vi "LoadState.vi"(3 "tabs":refnum<vi>, 4 "camera":string, 5 "file":path) -> ()   [LabVIEW 2010]
uses:
  <vilib>/addons/h5labview/H5F_mode.ctl
  <vilib>/addons/h5labview/polymorph/H5A_read_var.vi
  <vilib>/addons/h5labview/H5File.lvlib
  <vilib>/addons/h5labview/H5GroupObject.lvlib
  <vilib>/addons/h5labview/H5Attrib.lvlib
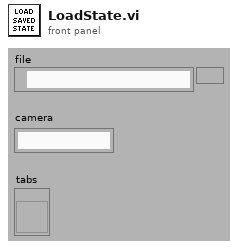
[diagram p1: front panel]
types:
  T1 = typedef "H5File.lvlib/H5F_mode.ctl" = enum16{"read-only", "read-write", "overwrite", "create new", "open or create"}
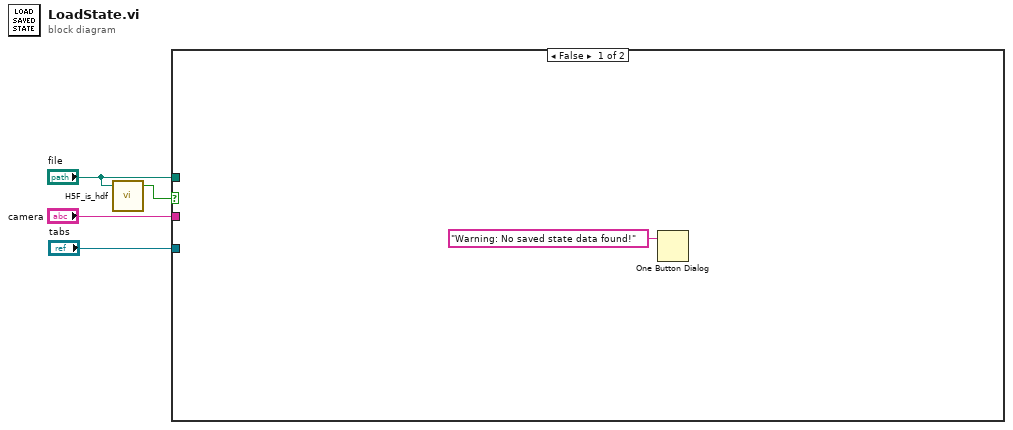
[diagram p0: block diagram]
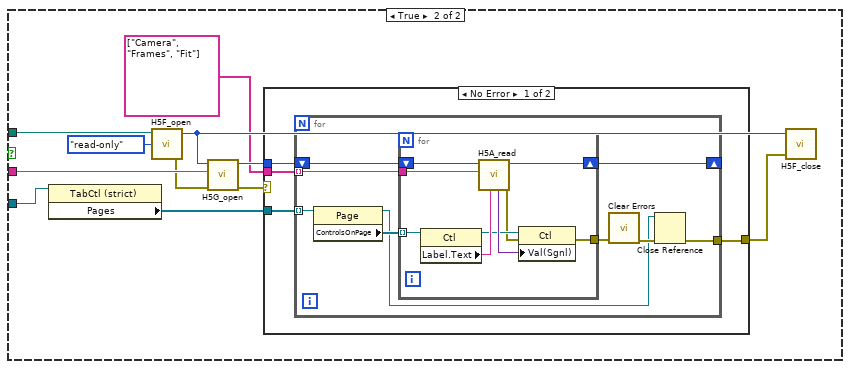
[diagram p2: hidden frame]
diagram:
  n1 = call <vilib>:"H5F_is_hdf.vi"("path"="file") -> ("valid"=w1:bool)  [unwired: 2 in, 2 out]
  n2 = case shown="False" w1 {
    tunnel: "camera" -> [_ w15]
    tunnel: "tabs" -> [_ w10]
    tunnel: "file" -> [_ w6]
    frame False {
      n3 = One Button Dialog(message="Warning: No saved state data found!") -> ()  [unwired: 1 in, 1 out]
    }
    frame True {
      n4 = property class="TabCtl (strict)"(reference=w10) -> ("Pages"=w9:refnum<vi>[])  [unwired: 1 in, 2 out]
      n5 = call <vilib>:"H5F_open.vi"("mode"=H5F_mode."read-only", "path"=w6) -> ("error out"=w13:errorcluster, "ref"=w14:i32)  [unwired: 2 in]
      n6 = call <vilib>:"H5G_open.vi"("error in (no error)"=w13, "name"=w15, "ref"=w14) -> ("error out"=w12:errorcluster, "group"=w11:i32)  [unwired: 3 in]
      n7 = case shown="No Error" w12 {
        tunnel: w11 -> [w20 _]
        tunnel: w9 -> [w19 _]
        tunnel: string[] ["Camera", "Frames", "Fit"] -> [w18 _]
        tunnel: [w17 _] -> w7
        frame No Error {
          n8 = for {
            tunnel: w19 -> [w29] mode=indexing
            shift-right: [w26] -> _
            shift-left: w20 -> [w27]
            tunnel: w18 -> [w25] mode=indexing
            tunnel: [w22] -> w17
            n9 = property class="Page"(reference=w29) -> (reference out=w21:refnum<vi>, "ControlsOnPage"=w28:refnum<vi>[])  [unwired: 1 in, 1 out]
            n10 = for {
              tunnel: w28 -> [w38] mode=indexing
              shift-right: [w33] -> w26
              shift-left: w27 -> [w37]
              tunnel: w25 -> [w32]
              tunnel: [w30] -> w24
              n11 = property class="Ctl"(reference=w38) -> (reference out=w34:refnum<vi>, "Label.Text"=w36:string)  [unwired: 1 in, 1 out]
              n12 = call-poly <vilib>:"H5A_read.vi"("attrib_name"=w36, "obj_name"=w32, "ref"=w37) -> ("error out"=w31:errorcluster, "ref out"=w33:i32, "value"=w35:variant)  [unwired: 4 in]
              n13 = property class="Ctl"(reference=w34, error in=w31, "Val(Sgnl)"=w35) -> (error out=w30:errorcluster)  [unwired: 1 out]
            }
            n14 = call <vilib>:"Clear Errors.vi"("error in (no error)"=w24) -> ("error out"=w23:errorcluster)  [unwired: 6 in]
            n15 = Close Reference(reference=w21, error in (no error)=w23) -> (error out=w22:errorcluster)
          }
        }
        frame Error {
        }
      }
      n16 = call <vilib>:"H5F_close.vi"("error in (no error)"=w7, "ref"=w14) -> ()  [unwired: 3 in, 1 out]
    }
  }
